vi "AddNew2DGraph.vi"(8 "error in (no error)":errorcluster caption="entrée d'erreur (pas d'erreur)", 9 "DataFileName":path, 10 "2DGphParam":T1={"ZDataIndex"=-1, "XParIndex"=-1, "YParIndex"=-1, "FillLineFirst"=FALSE, "2DGraphIndex"=0, "XParQ Ref"=refnum, "YParQ Ref"=refnum, "DataQRefs"=[], "CurveName"="", "XparInstrInd"=-1, "YparInstrInd"=-1, "Active"=FALSE}, 11 "Interface en entrée":refnum<class "Interface.lvclass"> caption="DNL_LabVIEW Object in") -> (0 "error out":errorcluster caption="sortie d'erreur", 1 "Graph":refnum<vi>, 2 "NewGraphInd":i32, 3 "Interface en sortie":refnum<class "Interface.lvclass"> caption="DNL_LabVIEW Object out", 4 "2DGraphQRef":refnum<queue>)   [LabVIEW 2019, in "Interface.lvclass"]
uses:
  Interface.lvclass
  2DGraphSetup.ctl
  Interface.lvclass/Interface.ctl
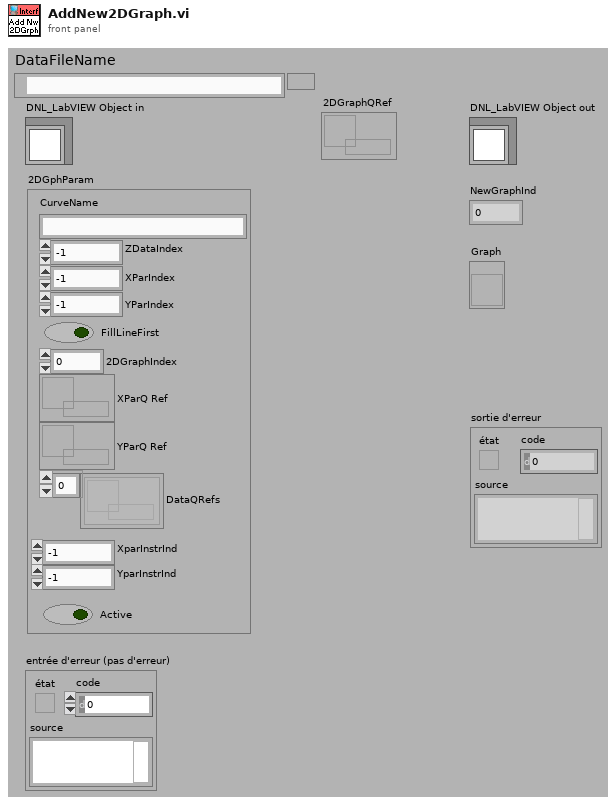
[diagram p1: front panel]
types:
  T1 = typedef "2DGraphSetup.ctl" = cluster{"ZDataIndex":i32, "XParIndex":i32, "YParIndex":i32, "FillLineFirst":bool, "2DGraphIndex":i32, "XParQ Ref":refnum<queue>, "YParQ Ref":refnum<queue>, "DataQRefs":refnum<queue>[], "CurveName":string, "XparInstrInd":i32, "YparInstrInd":i32, "Active":bool}
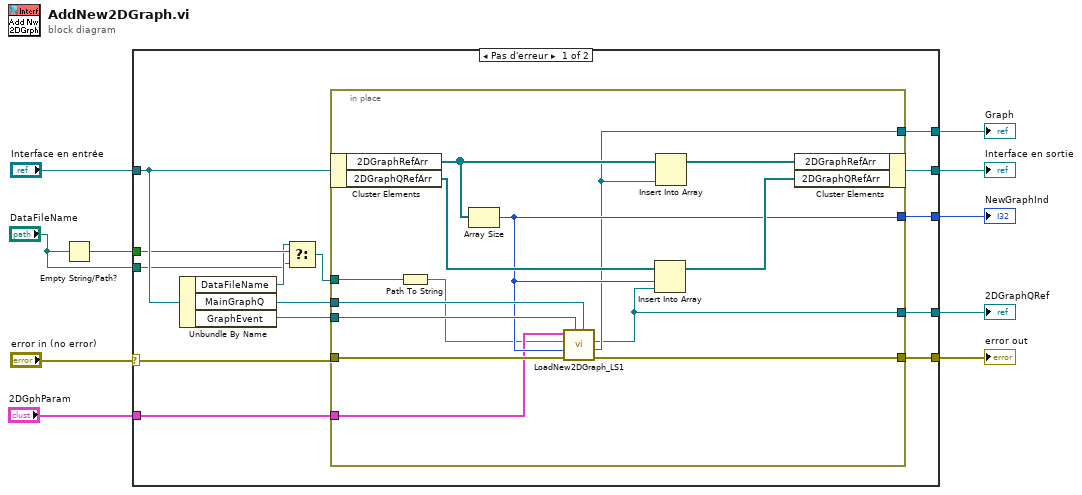
[diagram p0: block diagram]
diagram:
  n1 = Empty String/Path?(string/path="DataFileName") -> (empty?=w2:bool)
  n2 = case shown="Pas d'erreur" "error in (no error)" {
    selector: "error in (no error)" -> [w23 w40]
    tunnel: [w22 w40] -> w9
    tunnel: [w21 w39] -> w7
    tunnel: "Interface en entrée" -> [w20 w39]
    tunnel: [w24 _] -> w6
    tunnel: [w17 _] -> w5
    tunnel: [w16 _] -> w4
    tunnel: "2DGphParam" -> [w15 _]
    tunnel: w2 -> [w14 _]
    tunnel: "DataFileName" -> [w12 _]
    frame No Error {
      n3 = Unbundle By Name(w20) -> ("DataFileName"=w13:path, "MainGraphQ"=w19:refnum<queue>, "GraphEvent"=w18:refnum<user-event>)
      n4 = Select(t=w13, s=w14, f=w12) -> (s? t:f=w11:path)
      n5 = in-place {
        in-place-border: [w30] -> w24
        in-place-border: w23 -> [w33]
        in-place-border: [w38] -> w22
        in-place-border: w19 -> [w32]
        in-place-border: w18 -> [w31]
        in-place-border: [w29] -> w17
        in-place-border: [w28] -> w16
        in-place-border: w15 -> [w27]
        in-place-border: w11 -> [w25]
        n6 = in-place-cluster #1(w20) -> ("2DGraphRefArr"=w37:refnum<vi>[], "2DGraphQRefArr"=w35:refnum<queue>[])
        n7 = Path To String(path=w25) -> (string=w26:string)
        n8 = Array Size(array=w37) -> (size(s)=w30:i32)
        n9 = call "LoadNew2DGraph_LS1.vi"("MainGraphQ"=w32, "GraphEvent"=w31, "ErrorIn(No Error)"=w33, "GraphIndex"=w30, "Chemin"=w26, "2DGphParam"=w27) -> ("sortie d'erreur"=w38:errorcluster, "Graph"=w29:refnum<vi>, "2DGraphQRef"=w28:refnum<queue>)  [unwired: 3 in]
        n10 = Insert Into Array(array=w35, index=w30, new element=w28) -> (w34:refnum<queue>[])
        n11 = Insert Into Array(array=w37, new element=w29) -> (w36:refnum<vi>[])  [unwired: 1 in]
        n12 = in-place-cluster #1("2DGraphRefArr"=w36, "2DGraphQRefArr"=w34) -> (w21:refnum<class "Interface.lvclass">)
      }
    }
    frame Error {
    }
  }
  "error out" <- w9
  "Interface en sortie" <- w7
  "NewGraphInd" <- w6
  "Graph" <- w5
  "2DGraphQRef" <- w4
